vi "_Do Mass Range.vi"(2 "# of MR Offset":u16, 3 "Pause Time Offset":u16) -> ()   [LabVIEW 2012]
uses:
  <vilib>/rvi/DataTransferAndStorage/Container/Common/niFpgaContainerGetUniqueNameForEmu.vi
  <vilib>/rvi/Memory/Memory_Emulation/niFpgaMemoryEmulationCacheClearOnFirstRun.vi
  <vilib>/rvi/Memory/Memory_Emulation/nirvimemoryEmulationManagerCache_MakeExclusive.vi
  <vilib>/rvi/Memory/Memory_Emulation/niFpgaMemoryEmulationValidateCache.vi
  <vilib>/rvi/Memory/Memory_Emulation/nirvimemoryEmulationManagerCache_ReleaseExclusive.vi
  <vilib>/rvi/Memory/Memory_Emulation/nirvimemoryEmulationManagerCache_InsertValue.vi
  <vilib>/Utility/error.llb/Clear Errors.vi
  <vilib>/rvi/Memory/Memory_Emulation/nirvimemoryEmulationManagerCache_GetValue.vi
  Instance           1 22Saved   _Do Mass Range .vi
  Instance           2 22Saved   _Do Mass Range .vi
  <vilib>/rvi/Emulation/niFpgaSctlEmulationGetInTimedLoop.vi
  <vilib>/rvi/Memory/Memory_Emulation/nirvimemoryEmulationManagerCache_SetValue.vi
  <vilib>/rvi/Emulation/niFpgaSctlEmulationResourceMgr.vi
  <vilib>/rvi/interface/RandomDataEmulation/nirviRandomDataFPGAFIFO.vi
  <vilib>/rvi/interface/RandomDataEmulation/niFpgaRandomDataHandleErrors.vi
  <vilib>/rvi/DataTransferAndStorage/Container/XNode/niFpgaContainer.xnode
  <vilib>/rvi/Memory/Memory_Emulation/nirvimemoryEmulation.vi
  <vilib>/rvi/interface/RandomDataEmulation/nirviRandomDataFpgaReadWriteTemplate.vi
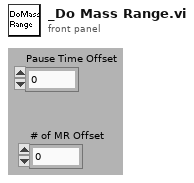
[diagram p1: front panel]
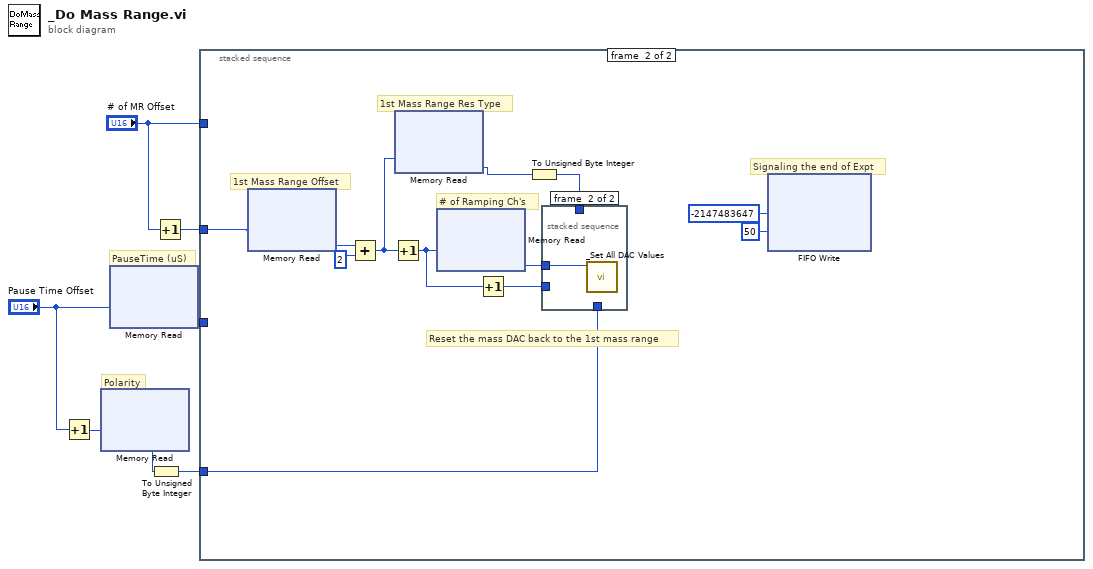
[diagram p0: block diagram]
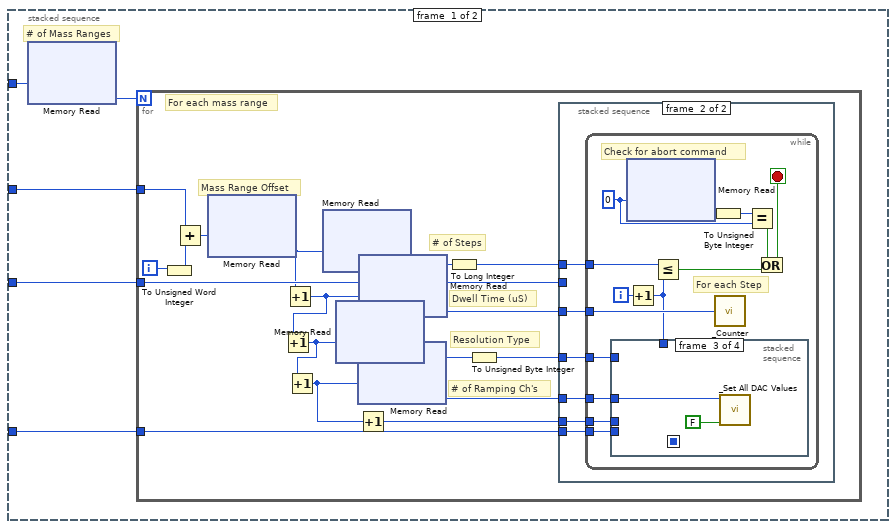
[diagram p2: hidden frame]
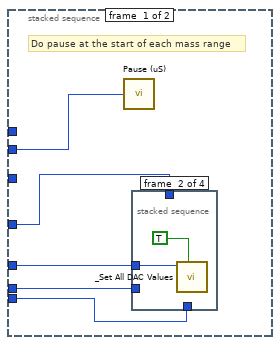
[diagram p3: hidden frame]
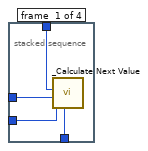
[diagram p4: hidden frame]
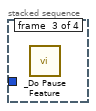
[diagram p5: hidden frame]
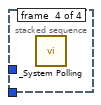
[diagram p6: hidden frame]
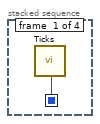
[diagram p7: hidden frame]
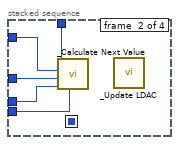
[diagram p8: hidden frame]
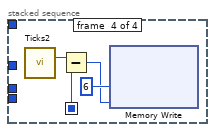
[diagram p9: hidden frame]
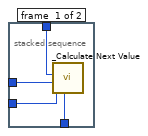
[diagram p10: hidden frame]
diagram:
  # "PauseTime (uS)"
  # "Polarity"
  n1 = Increment(x="Pause Time Offset") -> (x+1=w5:u16)
  n2 = xnode ("Memory Read")("Address"=w5) -> ("Data"=w2:u32)  [unwired: 1 in, 1 out]
  n3 = xnode ("Memory Read")("Address"="Pause Time Offset") -> ("Data"=w3:u32)  [unwired: 1 in, 1 out]
  n4 = To Unsigned Byte Integer(number=w2) -> (unsigned 8bit integer=w1:u8)
  n5 = Increment(x="# of MR Offset") -> (x+1=w6:u16)
  n6 = stacked-sequence {
    tunnel: "# of MR Offset" -> [w11 _]
    tunnel: w6 -> [w10 w74]
    tunnel: w1 -> [w9 w73]
    tunnel: w3 -> [w8 _]
    frame #0 {
      # "# of Mass Ranges"
      n7 = xnode ("Memory Read")("Address"=w11) -> ("Data"=w12:u32)  [unwired: 1 in, 1 out]
      n8 = for {
        N: w12 -> [_]
        tunnel: w10 -> [w28]
        tunnel: w9 -> [w27]
        tunnel: w8 -> [w26]
        i -> [w29]
        # "Resolution Type"
        # "Mass Range Offset"
        # "# of Ramping Ch's"
        # "Dwell Time (uS)"
        # "# of Steps"
        # "For each mass range"
        n9 = To Unsigned Word Integer(number=w29) -> (unsigned 16bit integer=w18:u16)
        n10 = Add(x=w28, y=w18) -> (x+y=w19:u16)
        n11 = xnode ("Memory Read")("Address"=w19) -> ("Data"=w17:u32)  [unwired: 1 in, 1 out]
        n12 = Increment(x=w17) -> (x+1=w16:u32)
        n13 = Increment(x=w16) -> (x+1=w15:u32)
        n14 = Increment(x=w15) -> (x+1=w23:u32)
        n15 = xnode ("Memory Read")("Address"=w17) -> ("Data"=w21:u32)  [unwired: 1 in, 1 out]
        n16 = xnode ("Memory Read")("Address"=w15) -> ("Data"=w14:u32)  [unwired: 1 in, 1 out]
        n17 = xnode ("Memory Read")("Address"=w23) -> ("Data"=w24:u32)  [unwired: 1 in, 1 out]
        n18 = Increment(x=w23) -> (x+1=w22:u32)
        n19 = xnode ("Memory Read")("Address"=w16) -> ("Data"=w25:u32)  [unwired: 1 in, 1 out]
        n20 = To Long Integer(number=w21) -> (32bit integer=w20:i32)
        n21 = To Unsigned Byte Integer(number=w14) -> (unsigned 8bit integer=w13:u8)
        n22 = stacked-sequence {
          tunnel: w25 -> [_ w46]
          tunnel: w24 -> [w33 w45]
          tunnel: w22 -> [w31 w44]
          tunnel: w20 -> [_ w43]
          tunnel: w13 -> [w30 w42]
          tunnel: w27 -> [w32 w41]
          tunnel: w26 -> [w34 _]
          frame #0 {
            # "Do pause at the start of each mass range"
            n23 = call "Pause (uS)"("Count(uSec)"=w34) -> ()  [unwired: 1 out]
            n24 = stacked-sequence {
              tunnel: w33 -> [w38 w40 _ _]
              tunnel: w31 -> [w37 _ _ _]
              tunnel: w30 -> [w36 _ _ _]
              tunnel: w32 -> [w35 _ _ _]
              frame #0 {
                n25 = call "_Calculate Next Value.vi"("Res Type"=w36, "# of Ramping Ch"=w38, "Parameter Offset"=w37, "Polarity"=w35) -> ()  [unwired: 1 in, 1 out]
              }
              frame #1 {
                n26 = call "_Set All DAC Values.vi"("Record Values (F)"=TRUE, "# of Active Channels"=w40) -> ()  [unwired: 7 in]
              }
              frame #2 {
                n27 = call "_Do Pause Feature.vi"() -> ()  [unwired: 6 in]
              }
              frame #3 {
                n28 = call "_System Polling.vi"() -> ()  [unwired: 6 out]
              }
            }
          }
          frame #1 {
            n29 = while {
              tunnel: w46 -> [w60]
              tunnel: w45 -> [w59]
              tunnel: w44 -> [w58]
              tunnel: w43 -> [w51]
              tunnel: w42 -> [w49]
              tunnel: w41 -> [w48]
              i -> [w50]
              stop <- w53 stop-if-true
              w55 = u8 0 ("Address")
              # "Check for abort command"
              # "For each Step"
              n30 = xnode ("Memory Read")("Address"=w55) -> ("Data"=w57:u32)  [unwired: 1 in, 1 out]
              n31 = Increment(x=w50) -> (x+1=w47:i32)
              n32 = stacked-sequence {
                seq-local: [w61 _ _ _] -> [_ _ _ w71]
                tunnel: w47 -> [_ w66 _ _]
                tunnel: w59 -> [_ w65 w68 _]
                tunnel: w58 -> [_ w64 _ _]
                tunnel: w49 -> [_ w63 _ _]
                tunnel: w48 -> [_ w62 _ _]
                frame #0 {
                  n33 = call "Ticks"() -> ("Tick Count(Ticks)"=w61:u16)
                }
                frame #1 {
                  n34 = call "_Calculate Next Value.vi"("Iteration#"=w66, "Res Type"=w63, "# of Ramping Ch"=w65, "Parameter Offset"=w64, "Polarity"=w62) -> ()  [unwired: 1 out]
                  n35 = call "_Update LDAC.vi"() -> ()  [unwired: 6 out]
                }
                frame #2 {
                  n36 = call "_Set All DAC Values.vi"("Load DAC(T)"=FALSE, "# of Active Channels"=w68) -> ()  [unwired: 7 in]
                }
                frame #3 {
                  n37 = call "Ticks2"() -> ("Tick Count(Ticks)"=w72:u16)
                  n38 = Subtract(x=w72, y=w71) -> (x-y=w69:u16)
                  n39 = xnode ("Memory Write")("Address"=u8 6, "Data"=w69) -> ()  [unwired: 1 in, 1 out]
                }
              }
              n40 = Less Or Equal?(x=w51, y=w47) -> (x <= y?=w52:bool)
              n41 = To Unsigned Byte Integer(number=w57) -> (unsigned 8bit integer=w56:u8)
              n42 = call "_Counter.vi"("Dwell (uS)"=w60) -> ()
              n43 = Equal?(x=w56, y=w55) -> (x = y?=w54:bool)
              n44 = Or(x=w54, y=w52) -> (x .or. y?=w53:bool)
            }
          }
        }
      }
    }
    frame #1 {
      # "Reset the mass DAC back to the 1st mass range"
      # "1st Mass Range Res Type"
      # "# of Ramping Ch's"
      # "1st Mass Range Offset"
      # "Signaling the end of Expt"
      n45 = xnode ("Memory Read")("Address"=w74) -> ("Data"=w78:u32)  [unwired: 1 in, 1 out]
      n46 = Add(x=w78, y=u8 2) -> (x+y=w76:u32)
      n47 = Increment(x=w76) -> (x+1=w75:u32)
      n48 = xnode ("Memory Read")("Address"=w76) -> ("Data"=w81:u32)  [unwired: 1 in, 1 out]
      n49 = xnode ("Memory Read")("Address"=w75) -> ("Data"=w80:u32)  [unwired: 1 in, 1 out]
      n50 = Increment(x=w75) -> (x+1=w79:u32)
      n51 = To Unsigned Byte Integer(number=w81) -> (unsigned 8bit integer=w82:u8)
      n52 = stacked-sequence {
        tunnel: w80 -> [w88 w89]
        tunnel: w79 -> [w87 _]
        tunnel: w82 -> [w86 _]
        tunnel: w73 -> [w85 _]
        frame #0 {
          n53 = call "_Calculate Next Value.vi"("Res Type"=w86, "# of Ramping Ch"=w88, "Parameter Offset"=w87, "Polarity"=w85) -> ()  [unwired: 1 in, 1 out]
        }
        frame #1 {
          n54 = call "_Set All DAC Values.vi"("# of Active Channels"=w89) -> ()  [unwired: 8 in]
        }
      }
      n55 = xnode ("FIFO Write")("Element"=-2147483647, "Timeout"=u8 50 ("Timeout (-1 for no timeout)")) -> ()  [unwired: 1 in, 2 out]
    }
  }
